vi "Process Telemetry Folder.vi"() -> ()   [LabVIEW 2014]
panel:
  in  "Output Folder":path=path "\\\\psf\\Dropbox/Formula Electric 2014-2015/Testing/02-21-15/Processed Data"
  in  "Input Folder":path=path "\\\\psf\\Dropbox/Formula Electric 2014-2015/Testing/02-21-15/Unprocessed Data"
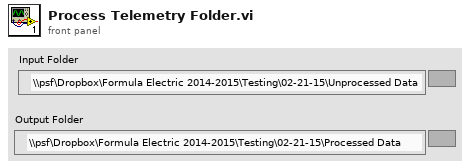
[diagram p1: front panel]
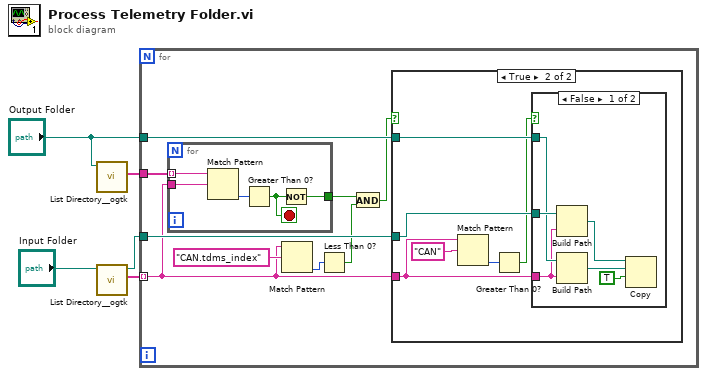
[diagram p0: block diagram]
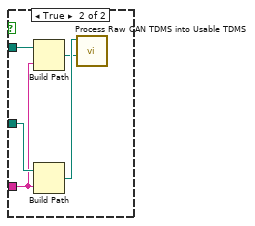
[diagram p3: hidden frame]
diagram:
  n1 = call <userlib>:"List Directory__ogtk.vi"("directory path"="Output Folder") -> ("file names"=w1:string[])  [unwired: 3 in, 3 out]
  n2 = call <userlib>:"List Directory__ogtk.vi"("directory path"="Input Folder") -> ("file names"=w4:string[], "dup directory path"=w3:path)  [unwired: 3 in, 2 out]
  n3 = for {
    tunnel: w4 -> [w6] mode=indexing
    tunnel: w3 -> [w14]
    tunnel: "Output Folder" -> [w13]
    tunnel: w1 -> [w8]
    n4 = for {
      tunnel: w8 -> [w19] mode=indexing
      tunnel: [w15] -> w7
      tunnel: w6 -> [w17]
      stop <- w16 stop-if-true
      n5 = Match Pattern(string=w19, regular expression=w17) -> (offset past match=w18:i32)  [unwired: 1 in, 3 out]
      n6 = Greater Than 0?(x=w18) -> (x > 0?=w16:bool)
      n7 = Not(x=w16) -> (.not. x?=w15:bool)
    }
    n8 = Match Pattern(string=w6, regular expression="CAN.tdms_index") -> (offset past match=w11:i32)  [unwired: 1 in, 3 out]
    n9 = Less Than 0?(x=w11) -> (x < 0?=w10:bool)
    n10 = And(x=w7, y=w10) -> (x .and. y?=w9:bool)
    n11 = case shown="True" w9 {
      tunnel: w14 -> [_ w25]
      tunnel: w13 -> [_ w24]
      tunnel: w6 -> [_ w23]
      frame False {
      }
      frame True {
        n12 = Match Pattern(string=w23, regular expression="CAN") -> (offset past match=w21:i32)  [unwired: 1 in, 3 out]
        n13 = Greater Than 0?(x=w21) -> (x > 0?=w20:bool)
        n14 = case shown="False" w20 {
          tunnel: w25 -> [w31 w36]
          tunnel: w24 -> [w30 w34]
          tunnel: w23 -> [w29 w33]
          frame False {
            n15 = Build Path(base path=w31, name or relative path=w29) -> (appended path=w28:path)
            n16 = Build Path(base path=w30, name or relative path=w29) -> (appended path=w27:path)
            n17 = Copy(9:TRUE ("overwrite (F)"), 10:w27, 11:w28) -> ()  [unwired: 2 in, 3 out]
          }
          frame True {
            n18 = Build Path(base path=w34, name or relative path=w33) -> (appended path=w32:path)
            n19 = Build Path(base path=w36, name or relative path=w33) -> (appended path=w35:path)
            n20 = call "Process Raw CAN TDMS into Usable TDMS.vi"("Destination"=w32, "Source"=w35) -> ()  [unwired: 10 in]
          }
        }
      }
    }
  }
